vi "TagDB Read States.vi"(8 "error in (no error)":errorcluster, 10 "StateNames":string[](array[string]), 11 "Refnum in":T1) -> (0 "error out":errorcluster, 2 "State":i32[](array[numeric]), 3 "Refnum out":T1)   [LabVIEW 2017, in "TagDB RefManager.lvlib"]
uses:
  TagDB RefManager.lvlib
  <userlib>/_NEVSTOP/TagDB/Typedef/TagDB.ctl
  171b747c-1da2-4803-875e-21dad1b386d6.vi
  d65ae9f0-a4bd-42b1-b196-be15abb22cd4.vi
  <userlib>/_NEVSTOP/TagDB/_Support/DataAccess/_NameCacher.vi
  <userlib>/_NEVSTOP/TagDB/_Support/DataAccess/TagDB Ref to DVR.vi
  <userlib>/_NEVSTOP/TagDB/_Support/URL/TRIM-BOTH-SPACE.vi
  <userlib>/_NEVSTOP/TagDB/_Support/Error/_[error50002]Invalid DataType.vi
  <userlib>/_NEVSTOP/TagDB/_Support/Error/_[error50000]Invalid DB REF.vi
  <vilib>/Utility/Data Type/NI_Data Type.lvlib
  <userlib>/_NEVSTOP/TagDB/TagDB.lvlib
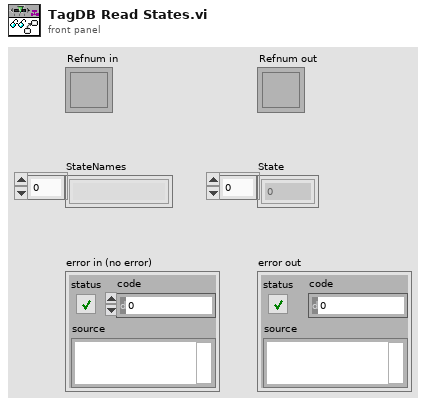
[diagram p1: front panel]
types:
  T1 = typedef "TagDB.lvlib/TagDB.ctl" = refnum<k1>
  T2 = typedef "NI_Data Type.lvlib/Data Type.ctl" = enum8{"Invalid Type", "Void", "I8", "I16", "I32", "I64", "U8", "U16", "U32", "U64", "Single Float", "Double Float", "Extended Float", "Single Complex", "Double Complex", "Extended Complex", "Enum U8", "Enum U16", "Enum U32", "Enum U64", "Single Float With Unit", "Double Float With Unit", "Extended Float With Unit", "Single Complex with Unit", "Double Complex with Unit", "Extended Complex with Unit", "Boolean", "String", "Path", "Picture", "Tag", "Array", "Cluster", "Variant", "LV Variant", "Waveform", "Timestamp", "Digital Waveform", "Digital Data", "ExpressData", "Refnum", "External Data", "VI", "Poly VI", "LabVIEW Class Instance", "Fixed Point"}
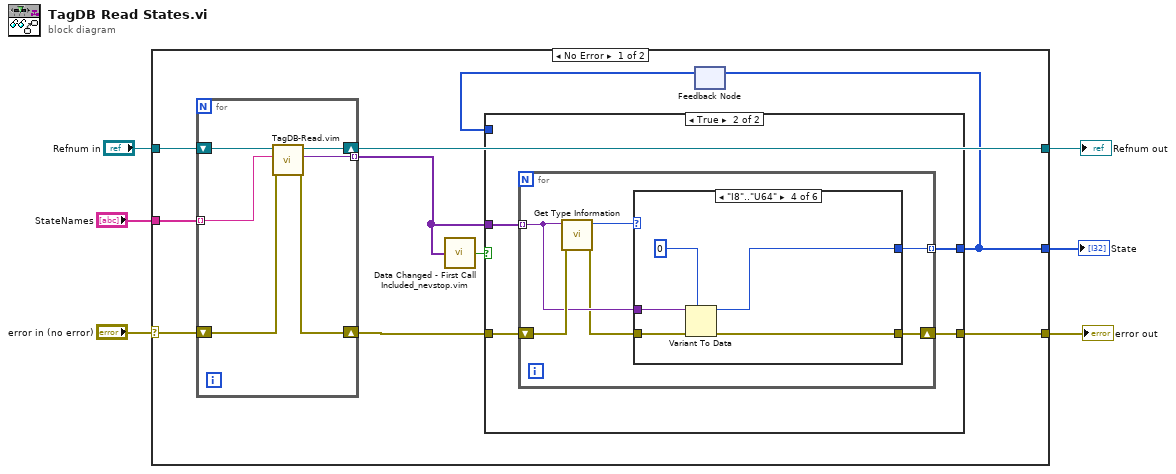
[diagram p0: block diagram]
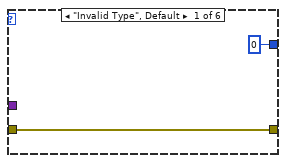
[diagram p3: hidden frame]
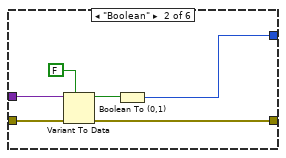
[diagram p4: hidden frame]
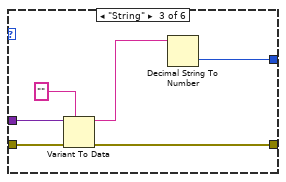
[diagram p5: hidden frame]
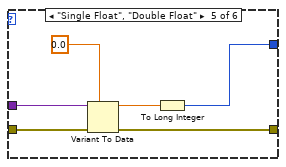
[diagram p6: hidden frame]
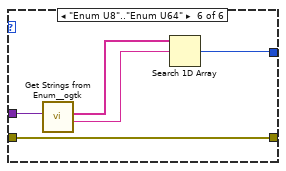
[diagram p7: hidden frame]
diagram:
  n1 = case shown="No Error" "error in (no error)" {
    selector: "error in (no error)" -> [w14 w66]
    tunnel: "Refnum in" -> [w16 w65]
    tunnel: "StateNames" -> [w15 _]
    tunnel: [w13 w65] -> w3
    tunnel: [w11 w66] -> w2
    tunnel: [w8 _] -> w1
    frame No Error {
      n2 = for {
        tunnel: w15 -> [w63] mode=indexing
        tunnel: [w59] -> w10 mode=indexing
        shift-right: [w61] -> w13
        shift-left: w16 -> [w64]
        shift-right: [w60] -> w12
        shift-left: w14 -> [w62]
        n3 = call "TagDB-Read.vim"("error in (no error)"=w62, "name"=w63, "TagDB"=w64) -> ("error out"=w60:errorcluster, "Value"=w59:variant, "TagDB(dup)"=w61:T1)  [unwired: 3 in, 3 out]
      }
      n4 = call "Data Changed - First Call Included_nevstop.vim"("Variant"=w10) -> ("Changed"=w9:bool)
      n5 = feedback #1() -> (w7:i32[])  [unwired: 1 in]
      n6 = case shown="True" w9 {
        tunnel: w12 -> [w18 w22]
        tunnel: [w18 w21] -> w11
        tunnel: [w17 w20] -> w8
        tunnel: w10 -> [_ w19]
        tunnel: w7 -> [w17 _]
        frame False {
        }
        frame True {
          n7 = for {
            tunnel: w19 -> [w26] mode=indexing
            tunnel: [w23] -> w20 mode=indexing
            shift-right: [w25] -> w21
            shift-left: w22 -> [w28]
            n8 = call <vilib>:"Get Type Information.vi"("error in (no error)"=w28, "Variant"=w26) -> ("error out"=w24:errorcluster, "Type"=w27:T2)  [unwired: 5 in, 3 out]
            n9 = case shown="\"I8\"..\"U64\"" w27 {
              tunnel: w26 -> [_ w34 w40 w46 w52 w57]
              tunnel: [w29 w35 w41 w44 w50 w58] -> w25
              tunnel: w24 -> [w29 w36 w42 w47 w53 w58]
              tunnel: [0 ("index of element") w31 w37 w43 w48 w56] -> w23
              frame "Invalid Type", Default {
              }
              frame "Boolean" {
                n10 = Variant To Data(error in=w36, type=FALSE, Variant=w34) -> (data=w32:bool, error out=w35:errorcluster)
                n11 = Boolean To (0,1)(Boolean=w32) -> (0, 1=w31:i16)
              }
              frame "String" {
                n12 = Variant To Data(error in=w42, type="", Variant=w40) -> (data=w38:string, error out=w41:errorcluster)
                n13 = Decimal String To Number(string=w38) -> (number=w37:i32)  [unwired: 2 in, 1 out]
              }
              frame "I8".."U64" {
                n14 = Variant To Data(error in=w47, type=0, Variant=w46) -> (data=w43:i32, error out=w44:errorcluster)
              }
              frame "Single Float", "Double Float" {
                n15 = Variant To Data(error in=w53, type=sgl 0.0, Variant=w52) -> (data=w49:sgl, error out=w50:errorcluster)
                n16 = To Long Integer(number=w49) -> (32bit integer=w48:i32)
              }
              frame "Enum U8".."Enum U64" {
                n17 = call <userlib>:"Get Strings from Enum__ogtk.vi"("Enum"=w57) -> ("String Value"=w54:string, "Enum Strings"=w55:string[])  [unwired: 7 in, 2 out]
                n18 = Search 1D Array(1D array=w55, element=w54) -> (index of element=w56:i32)  [unwired: 1 in]
              }
            }
          }
        }
      }
      n19 = feedback-in #1(w8) -> ()
    }
    frame Error {
    }
  }
  "error out" <- w2
  "Refnum out" <- w3
  "State" <- w1
